vi "Module.LaunchVI.vi"(4 "Init Ctrl Values":cluster{"Ctrl Name":string, "Value":variant}[](array[cluster]), 5 "Index":i32, 6 "Working Dirs":T1, 7 "Reentrant":bool, 8 "error in":errorcluster, 9 "Q Name":string, 10 "VI Path":path, 11 "Parent Q":refnum<queue>) -> (0 "error out":errorcluster, 2 "Name Out":string, 3 "reference out":refnum<vi>)   [LabVIEW 2024, in "EQMF.lvlib" / "Module Utils.lvlib"]
uses:
  Module Utils.lvlib
  Module.Working Dirs.ctl
  Queues/Q.Element.ctl
  Module Config.ctl
  Queues/Queue Utils.lvlib
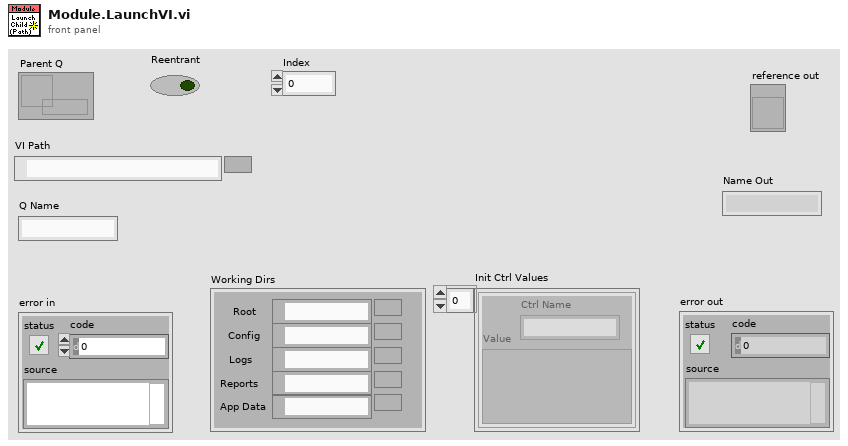
[diagram p1: front panel]
types:
  T1 = typedef "EQMF.lvlib/Module Utils.lvlib/Module.Working Dirs.ctl" = cluster{"Root":path, "Config":path, "Logs":path, "Reports":path, "App Data":path}
  T2 = typedef "EQMF.lvlib/Queue Utils.lvlib/Q.Element.ctl" = cluster{"Cmd":string, "Sub":string, "Data1":variant, "Data2":variant}
  T3 = typedef "EQMF.lvlib/Module Utils.lvlib/Module Config.ctl" = cluster{"Name":string, "Parent Q":refnum<queue>, "Is Child?":bool, "Index":i32, "Dirs":T1, "Simulate":bool, "SimCtrl":refnum<vi>}
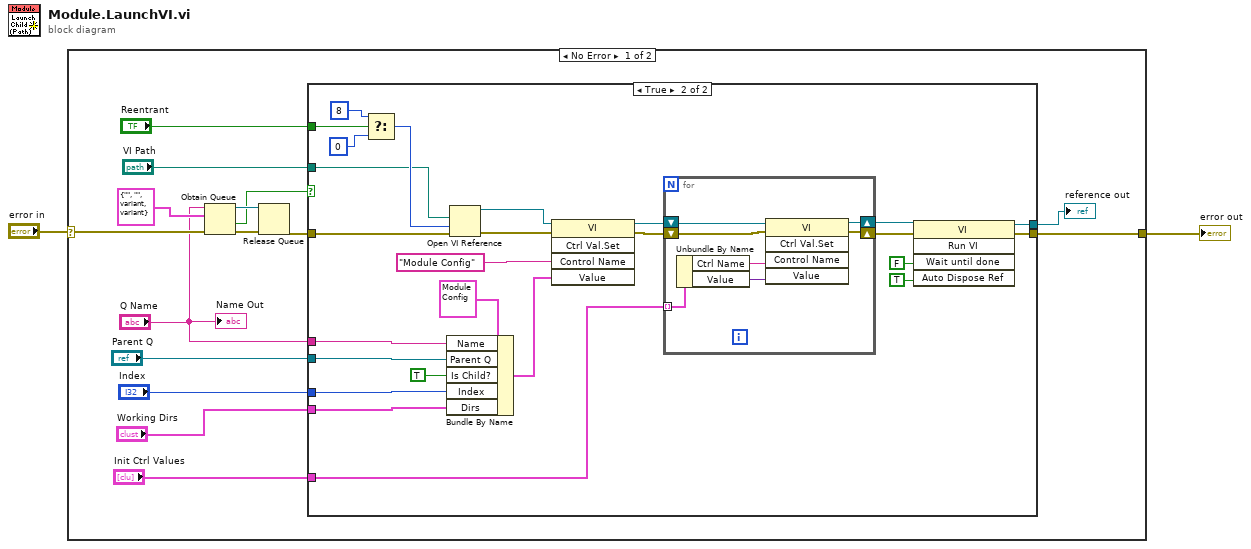
[diagram p0: block diagram]
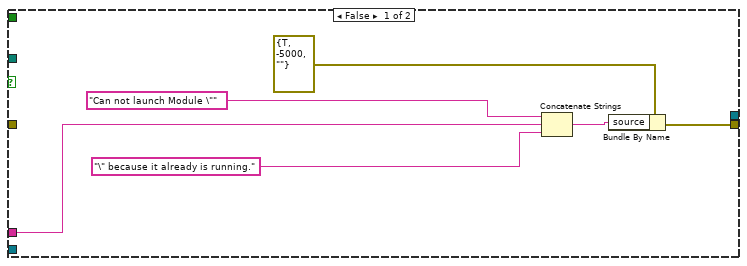
[diagram p2: hidden frame]
diagram:
  n1 = case shown="No Error" "error in" {
    selector: "error in" -> [w7 w56]
    tunnel: [w8 w56] -> w2
    frame No Error {
      n2 = Obtain Queue(name (unnamed)="Q Name", element data type=T2 {"Cmd"="", "Sub"="", "Data1"=variant, "Data2"=variant} ("MainQ.Element"), error in (no error)=w7) -> (queue out=w10:refnum<queue>, created new?=w9:bool, error out=w12:errorcluster)  [unwired: 2 in]
      n3 = Release Queue(queue=w10, error in (no error)=w12) -> (error out=w11:errorcluster)  [unwired: 1 in, 2 out]
      n4 = case shown="True" w9 {
        tunnel: "VI Path" -> [_ w45]
        tunnel: w11 -> [_ w41]
        tunnel: "Reentrant" -> [_ w40]
        tunnel: "Q Name" -> [w21 w37]
        tunnel: "Parent Q" -> [_ w36]
        tunnel: "Index" -> [_ w34]
        tunnel: "Working Dirs" -> [_ w33]
        tunnel: [w20 w32] -> w8
        tunnel: [_ w31] -> w5
        tunnel: "Init Ctrl Values" -> [_ w24]
        frame False {
          n5 = Concatenate Strings("Can not launch Module \"", w21, "\" because it already is running.") -> (w18:string)
          n6 = Bundle By Name(cluster=errorcluster {"status"=TRUE, "code"=-5000, "source"=""} ("error constant"), "source"=w18) -> (w20:errorcluster)
        }
        frame True {
          n7 = Select(t=8 ("options"), s=w40, f=0 ("options")) -> (s? t:f=w46:i32)
          n8 = Bundle By Name(cluster=T3 {"Name"="", "Parent Q"=refnum, "Is Child?"=FALSE, "Index"=0, "Dirs"={"Root"=path "", "Config"=path "", "Logs"=path "", "Reports"=path "", "App Data"=path ""}, "Simulate"=FALSE, "SimCtrl"=refnum}, "Name"=w37, "Parent Q"=w36, "Is Child?"=TRUE ("Child"), "Index"=w34, "Dirs"=w33) -> (w38:T3)
          n9 = Open VI Reference(vi path=w45, options=w46, error in (no error)=w41) -> (vi reference=w30:refnum<vi>, error out=w29:errorcluster)  [unwired: 3 in]
          n10 = invoke class="VI" method="Ctrl Val.Set"(reference=w30, error in=w29, "Control Name"="Module Config", "Value"=w38) -> (reference out=w28:refnum<vi>, error out=w27:errorcluster)  [unwired: 1 in, 3 out]
          n11 = for {
            shift-right: [w53] -> w26
            shift-left: w28 -> [w55]
            shift-right: [w52] -> w25
            shift-left: w27 -> [w54]
            tunnel: w24 -> [w51] mode=indexing
            n12 = Unbundle By Name(w51) -> ("Ctrl Name"=w49:string, "Value"=w50:variant)
            n13 = invoke class="VI" method="Ctrl Val.Set"(reference=w55, error in=w54, "Control Name"=w49, "Value"=w50) -> (reference out=w53:refnum<vi>, error out=w52:errorcluster)  [unwired: 1 in, 3 out]
          }
          n14 = invoke class="VI" method="Run VI"(reference=w26, error in=w25, "Wait until done"=FALSE ("Wait Until Done"), "Auto Dispose Ref"=TRUE ("Auto Dispose Reference")) -> (reference out=w31:refnum<vi>, error out=w32:errorcluster)  [unwired: 1 in, 3 out]
        }
      }
      "reference out" <- w5
      "Name Out" <- "Q Name"
    }
    frame Error {
    }
  }
  "error out" <- w2
